vi "Communication delay and error simulator.vi"(0 "VISA name in":refnum<visa-resource-name>, 1 "Modem dealay sim":bool, 5 "Transmitt string":string, 7 "Sim baud Tx":u16, 9 "Bit Error fraction Tx":dbl, 11 "error in":errorcluster) -> (4 "VISA name out":refnum<visa-resource-name>, 6 "string with bit errors":string, 15 "error out":errorcluster)   [LabVIEW 2011]
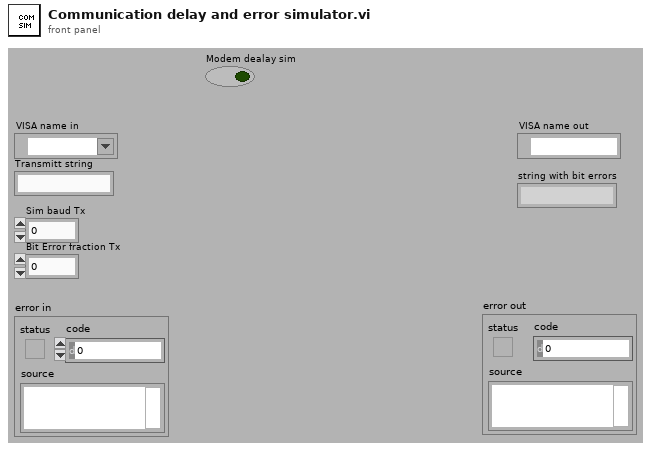
[diagram p1: front panel]
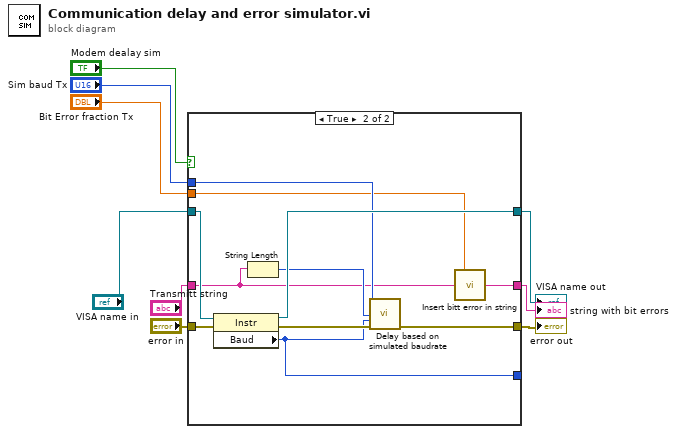
[diagram p0: block diagram]
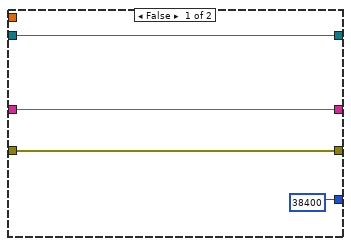
[diagram p2: hidden frame]
diagram:
  n1 = case shown="True" "Modem dealay sim" {
    tunnel: [w13 w20] -> w1
    tunnel: "error in" -> [w13 w22]
    tunnel: "Sim baud Tx" -> [_ w21]
    tunnel: "VISA name in" -> [w12 w24]
    tunnel: [w12 w23] -> w6
    tunnel: "Transmitt string" -> [w10 w16]
    tunnel: [w10 w15] -> w8
    tunnel: "Bit Error fraction Tx" -> [_ w17]
    tunnel: [u32 38400 ("Baud") w14] -> _
    frame False {
    }
    frame True {
      n2 = property class="Instr"(reference=w24, error in=w22) -> (reference out=w23:refnum<visa-resource-name>, error out=w19:errorcluster, "Baud"=w14:u32)
      n3 = String Length(string=w16) -> (length=w18:i32)
      n4 = call "Delay based on simulated baudrate.vi"("Budrate to simulate"=w21, "Number of bytes"=w18, "Line Baudrate"=w14, "error in"=w19) -> ("error out"=w20:errorcluster)  [unwired: 11 in]
      n5 = call "Insert bitt error in string.vi"("Fault(fraction = 0)"=w17, "Transmitt string"=w16) -> ("string with bit errors"=w15:string)  [unwired: 13 in]
    }
  }
  "string with bit errors" <- w8
  "VISA name out" <- w6
  "error out" <- w1
